vi "Receive Omni Packet.vi"   [LabVIEW 2013]
uses:
  Common Code/Dashboard UDP/Omni Packet.ctl
  Common Code/Dashboard UDP Packet.ctl
  Common Code/Dashboard UDP/Camera Controls.ctl
  Common Code/Dashboard UDP/Gyro Controls.ctl
  Common Code/Dashboard UDP/PID Params.ctl
  Common Code/Dashboard UDP/Encoder Controls.ctl
  Common Code/Dashboard UDP/Auto Shift Controls.ctl
  Common Code/Dashboard UDP/Auton Controls.ctl
  Common Code/Dashboard UDP/Shooter Controls.ctl
  Common Code/Dashboard UDP/Roller Controls.ctl
  Common Code/Vision Mode.ctl
  Common Code/Dashboard UDP/Fieldcentric Controls.ctl
  Common Code/Dashboard UDP/Roll Maneuver.ctl
  Robot Global Data.vi
types:
  T1 = typedef "Omni Packet.ctl" = cluster{"Type":i32, "data string":string}
  T2 = typedef "Dashboard UDP Packet.ctl" = cluster{"Camera":T3, "Gyro":T4, "Encoder":T6, "Auto Shift":T7, "Auton":T8, "Drive/Ramp X":dbl, "Drive/Ramp Y":dbl, "Drive/Battery Cutoff":dbl, "Pressure/Compressor Min Voltage":dbl, "Pressure/Compressor Delay":dbl, "Controller/Strafe Correction":bool, "Shooter":T9, "Rollers":T10, "Abort":bool, "Finish":bool, "IR Halo Sustain Time":dbl, "Disable Compressor":bool, "Center Omni Drive Delay":i32, "Vision Mode":T11, "Radius Throttle":bool, "Fieldcentric":T12, "Roll":T13, "Stick Deadband":dbl}
  T3 = typedef "Camera Controls.ctl" = cluster{"Camera/View Angle X":dbl, "Camera/Goal Track Timeout":dbl, "Camera/View Angle Y":dbl, "Camera/Goal Exposure":dbl, "Camera/Vision Receive Timeout":dbl, "Camera/Offset 1":dbl, "Camera/Offset 2":dbl}
  T4 = typedef "Gyro Controls.ctl" = cluster{"Gyro/Angle Tolerance":dbl, "Gyro/Steer Closeness Threshold":dbl, "Steer PID":T5, "Steer Close PID":T5}
  T5 = typedef "PID Params.ctl" = cluster{"max":dbl, "min":dbl, "P":dbl, "I":dbl, "D":dbl}
  T6 = typedef "Encoder Controls.ctl" = cluster{"Encoders/Reset":bool, "Encoders/Omni Constant":dbl, "Encoders/Omni Tick Constant":dbl, "Encoders/Left Constant":dbl, "Encoders/Right Constant":dbl, "Encoders/Right Tick Constant":dbl}
  T7 = typedef "Auto Shift Controls.ctl" = cluster{"AutoShift/Upshift Throttle Accel":dbl, "AutoShift/Speed Threshold":dbl, "AutoShift/Upshift Throttle":dbl, "AutoShift/Upshift Accel":dbl, "AutoShift/Downshift Accel":dbl, "AutoShift/Downshift Throttle":dbl, "AutoShift/Delay":dbl, "AutoShift/Enabled":bool}
  T8 = typedef "Auton Controls.ctl" = cluster{"Auton/Left Shoot X-Coord":dbl, "Auton/Right Shoot X-Coord":dbl, "DistDrive/Distance Stop Threshold":dbl, "DistDrive/Max Stop Speed":dbl, "Auton/Back Piston Time":dbl, "Auton/Manual Hot":bool, "Auton/Manual Hot Right":bool, "Default X PID":T5, "Default Y PID":T5, "Half Over Delay":dbl}
  T9 = typedef "Shooter Controls.ctl" = cluster{"Shooter/Reset Time":dbl, "Shooter/Release Delay":dbl, "Shooter/Pressure Steady Time":dbl, "Shooter/Misfire Delay":dbl, "Shooter/Ball Settle Time":dbl, "Shooter/Line IR Delay":dbl, "Pressure/Upper PSI Time":dbl, "Pressure/Lower PSI Time":dbl, "Shooter/Punch Delay":dbl, "Shooter/Target Pressure":dbl, "Pressure/Line B":dbl, "Pressure/Line M":dbl, "Pressure/Shooter M":dbl, "Pressure/Shooter B":dbl, "Halo Time":dbl, "Soft Release Delay":dbl, "Soft Unpin Delay":dbl, "Soft Shoot Delay":dbl, "Toss Release Time":dbl}
  T10 = typedef "Roller Controls.ctl" = cluster{"Roller/Load IRs Verify Time":dbl, "Roller/Center IR Latch Time":dbl, "Roller/Speed Front":dbl, "Roller/Speed Back":dbl, "Roller/Entry Timeout":dbl, "Roller/To Center Timeout":dbl, "Roller/Sustain Time":dbl, "Roller/Verify Center Time":dbl}
  T11 = typedef "Vision Mode.ctl" = enum16{"Normal", "Extreme Left", "Extreme Right"}
  T12 = typedef "Fieldcentric Controls.ctl" = cluster{"Relative Angle":bool, "Point Robot":bool, "X/Y ratio low":dbl, "Steering Gain":dbl, "Force Omni Down":bool, "Enable":bool, "X/Y ratio high":dbl}
  T13 = typedef "Roll Maneuver.ctl" = cluster{"X 1":dbl, "Y 1":dbl, "Y 2":dbl, "X 2":dbl, "Y 3":dbl, "X 3":dbl, "Time 1":i32, "Time 2":i32, "Time 3":i32, "Angle Start":dbl, "Angle End":dbl, "Angle Linearity":dbl}
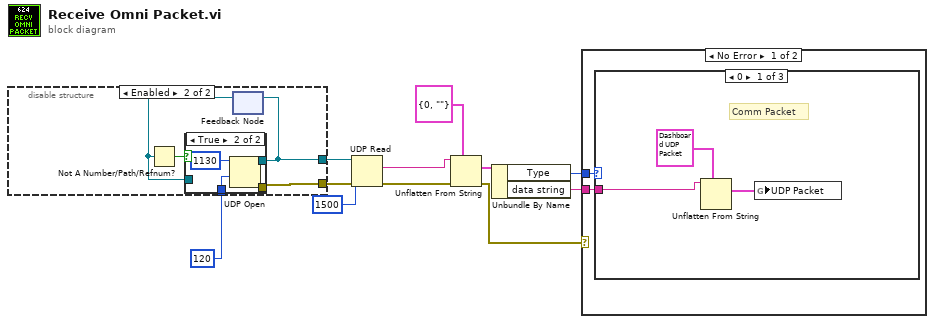
[diagram p0: block diagram]
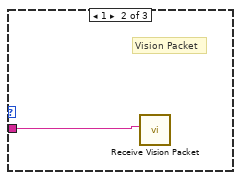
[diagram p2: hidden frame]
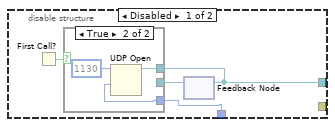
[diagram p5: hidden frame]
diagram:
  n1 = disable-structure shown="Enabled" {
    disable-tunnel: [w14 w23] -> w11
    disable-tunnel: [_ w24] -> w3
    disable-tunnel: 120 ("Numeric") -> [w12 w20]
    frame Disabled {
      n2 = First Call?() -> (First Call?: T/F=w15:bool)
      n3 = feedback #1() -> (w13:refnum<k16>)  [unwired: 1 in]
      n4 = case shown="True" w15 {
        tunnel: [w16 w18] -> w14
        tunnel: w13 -> [w16 _]
        tunnel: w12 -> [_ w17]
        frame False {
        }
        frame True {
          n5 = UDP Open(9:w17, 11:u16 1130 ("port")) -> (port=w18:refnum<k16>)  [unwired: 3 in, 2 out]
        }
      }
      n6 = feedback-in #1(w14) -> ()
    }
    frame Enabled {
      n7 = feedback #2() -> (w21:refnum<k16>)  [unwired: 1 in]
      n8 = Not A Number/Path/Refnum?(number/path/refnum=w21) -> (NaN/Path/Refnum?=w22:bool)
      n9 = case shown="True" w22 {
        tunnel: [_ w28] -> w24
        tunnel: [w25 w27] -> w23
        tunnel: w21 -> [w25 _]
        tunnel: w20 -> [_ w26]
        frame False {
        }
        frame True {
          n10 = UDP Open(9:w26, 11:u16 1130 ("port")) -> (port=w27:refnum<k16>, 0:w28:errorcluster)  [unwired: 3 in, 1 out]
        }
      }
      n11 = feedback-in #2(w23) -> ()
    }
  }
  n12 = UDP Read(connection ID=w11, max size (548)=1500, 8:w3) -> (data out=w8:string, error out=w7:errorcluster)  [unwired: 1 in, 3 out]
  n13 = Unflatten From String(type=T1 {"Type"=0, "data string"=""} ("OmniPacket"), binary string=w8, error in (no error)=w7) -> (value=w6:T1, error out=w2:errorcluster)  [unwired: 2 in, 1 out]
  n14 = Unbundle By Name(w6) -> ("Type"=w5:i32, "data string"=w4:string)
  n15 = case shown="No Error" w2 {
    tunnel: w5 -> [w31 _]
    tunnel: w4 -> [w30 _]
    frame No Error {
      n16 = case shown="0" w31 {
        tunnel: w30 -> [w33 w35 _]
        frame 0 {
          # "Comm Packet"
          n17 = Unflatten From String(type=T2 {"Camera"={"Camera/View Angle X"=-1.0, "Camera/Goal Track Timeout"=-1.0, "Camera/View Angle Y"=-1.0, "Camera/Goal Exposure"=-1.0, "Camera/Vision Receive Timeout"=-1.0, "Camera/Offset 1"=-1.0, "Camera/Offset 2"=-1.0}, "Gyro"={"Gyro/Angle Tolerance"=-1.0, "Gyro/Steer Closeness Threshold"=-1.0, "Steer PID"={"max"=-1.0, "min"=-1.0, "P"=-1.0, "I"=-1.0, "D"=-1.0}, "Steer Close PID"={"max"=-1.0, "min"=-1.0, "P"=-1.0, "I"=-1.0, "D"=-1.0}}, "Encoder"={"Encoders/Reset"=FALSE, "Encoders/Omni Constant"=-1.0, "Encoders/Omni Tick Constant"=-1.0, "Encoders/Left Constant"=-1.0, "Encoders/Right Constant"=-1.0, "Encoders/Right Tick Constant"=-1.0}, "Auto Shift"={"AutoShift/Upshift Throttle Accel"=-1.0, "AutoShift/Speed Threshold"=-1.0, "AutoShift/Upshift Throttle"=-1.0, "AutoShift/Upshift Accel"=-1.0, "AutoShift/Downshift Accel"=-1.0, "AutoShift/Downshift Throttle"=-1.0, "AutoShift/Delay"=-1.0, "AutoShift/Enabled"=FALSE}, "Auton"={"Auton/Left Shoot X-Coord"=-1.0, "Auton/Right Shoot X-Coord"=-1.0, "DistDrive/Distance Stop Threshold"=0.0, "DistDrive/Max Stop Speed"=0.0, "Auton/Back Piston Time"=-1.0, "Auton/Manual Hot"=FALSE, "Auton/Manual Hot Right"=FALSE, "Default X PID"={"max"=-1.0, "min"=-1.0, "P"=-1.0, "I"=-1.0, "D"=-1.0}, "Default Y PID"={"max"=-1.0, "min"=-1.0, "P"=-1.0, "I"=-1.0, "D"=-1.0}, "Half Over Delay"=0.0}, "Drive/Ramp X"=-1.0, "Drive/Ramp Y"=-1.0, "Drive/Battery Cutoff"=-1.0, "Pressure/Compressor Min Voltage"=-1.0, "Pressure/Compressor Delay"=-1.0, "Controller/Strafe Correction"=FALSE, "Shooter"={"Shooter/Reset Time"=-1.0, "Shooter/Release Delay"=-1.0, "Shooter/Pressure Steady Time"=-1.0, "Shooter/Misfire Delay"=-1.0, "Shooter/Ball Settle Time"=-1.0, "Shooter/Line IR Delay"=-1.0, "Pressure/Upper PSI Time"=-1.0, "Pressure/Lower PSI Time"=-1.0, "Shooter/Punch Delay"=-1.0, "Shooter/Target Pressure"=-1.0, "Pressure/Line B"=-1.0, "Pressure/Line M"=-1.0, "Pressure/Shooter M"=-1.0, "Pressure/Shooter B"=-1.0, "Halo Time"=0.0, "Soft Release Delay"=0.0, "Soft Unpin Delay"=0.0, "Soft Shoot Delay"=0.0, "Toss Release Time"=0.0}, "Rollers"={"Roller/Load IRs Verify Time"=-1.0, "Roller/Center IR Latch Time"=-1.0, "Roller/Speed Front"=-1.0, "Roller/Speed Back"=-1.0, "Roller/Entry Timeout"=-1.0, "Roller/To Center Timeout"=-1.0, "Roller/Sustain Time"=-1.0, "Roller/Verify Center Time"=-1.0}, "Abort"=FALSE, "Finish"=FALSE, "IR Halo Sustain Time"=0.0, "Disable Compressor"=FALSE, "Center Omni Drive Delay"=0, "Vision Mode"=enum."Normal", "Radius Throttle"=FALSE, "Fieldcentric"={"Relative Angle"=FALSE, "Point Robot"=FALSE, "X/Y ratio low"=0.0, "Steering Gain"=0.0, "Force Omni Down"=FALSE, "Enable"=FALSE, "X/Y ratio high"=0.0}, "Roll"={"X 1"=0.0, "Y 1"=0.0, "Y 2"=0.0, "X 2"=0.0, "Y 3"=0.0, "X 3"=0.0, "Time 1"=0, "Time 2"=0, "Time 3"=0, "Angle Start"=0.0, "Angle End"=0.0, "Angle Linearity"=0.0}, "Stick Deadband"=0.0} ("UDP Packet"), binary string=w33) -> (value=w32:T2)  [unwired: 3 in, 2 out]
          n18 = global write "Robot Global Data.vi" "UDP Packet"(w32) -> ()
        }
        frame 1 {
          # "Vision Packet"
          n19 = call "Receive Vision Packet.vi"("Packet"=w35) -> ()  [unwired: 11 in]
        }
        frame Default {
        }
      }
    }
    frame Error {
    }
  }
